vi "Stop.vi"() -> ()   [LabVIEW 2017]
panel:
  out "Stop":bool
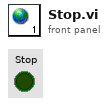
[diagram p1: front panel]
diagram:
